vi "set_counter_settings.vi"(8 "error in (no error)":errorcluster, 10 "counter":T1, 11 "GenericSignalWriter in":refnum<class "GenericSignalWriter.lvclass">) -> (0 "error out":errorcluster, 3 "GenericSignalWriter out":refnum<class "GenericSignalWriter.lvclass">)   [LabVIEW 2010, in "GenericSignalWriter.lvclass"]
uses:
  GenericSignalWriter.lvclass
  common/clusters/counter_settings_cluster.ctl
  GenericSignalWriter.lvclass/GenericSignalWriter.ctl
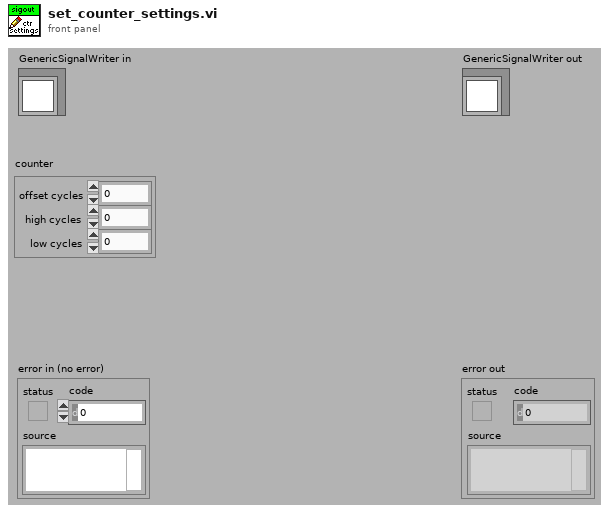
[diagram p1: front panel]
types:
  T1 = typedef "counter_settings_cluster.ctl" = cluster{"offset cycles":i32, "high cycles":i32, "low cycles":i32}
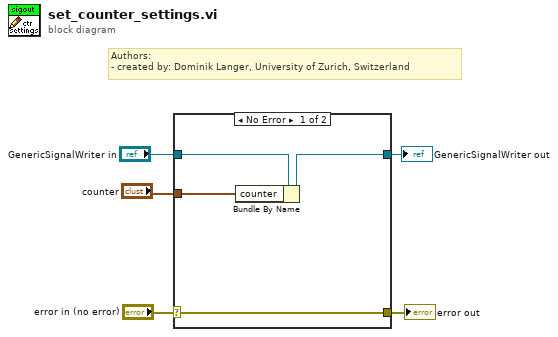
[diagram p0: block diagram]
diagram:
  # "Authors: \n- created by: Dominik Langer, University of Zurich, Switzerland"
  n1 = case shown="No Error" "error in (no error)" {
    selector: "error in (no error)" -> [w9 w11]
    tunnel: [w9 w11] -> w4
    tunnel: [w6 w10] -> w2
    tunnel: "GenericSignalWriter in" -> [w7 w10]
    tunnel: "counter" -> [w8 _]
    frame No Error {
      n2 = Bundle By Name(cluster=w7, "counter"=w8) -> (w6:refnum<class "GenericSignalWriter.lvclass">)
    }
    frame Error {
    }
  }
  "error out" <- w4
  "GenericSignalWriter out" <- w2
